vi "Joystick ReMap.vi"(2 "Deadband Size":dbl=0.02 min=-1.0 max=1.0 step=0.01, 3 "Raw Value":dbl) -> (0 "Modified Value (x^2)":dbl, 1 "Modified Value":dbl)   [LabVIEW 2014]
panel:
  # "The value entered here will be applied to both positive\nand negative values, so in a literal sense it is 1/2 the deadband\nsize, centered about zero."
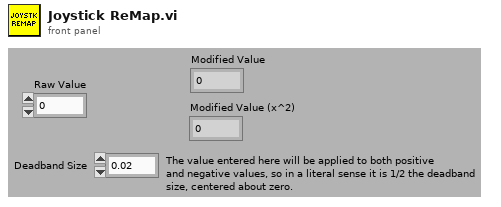
[diagram p1: front panel]
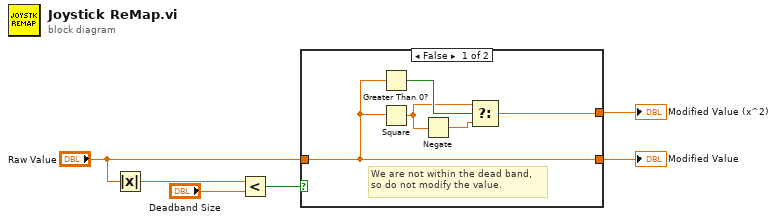
[diagram p0: block diagram]
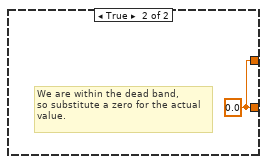
[diagram p2: hidden frame]
diagram:
  n1 = Absolute Value(x="Raw Value") -> (abs(x)=w5:dbl)
  n2 = Less?(x=w5, y="Deadband Size") -> (x < y?=w4:bool)
  n3 = case shown="False" w4 {
    tunnel: [w11 w12] -> w3
    tunnel: "Raw Value" -> [w11 _]
    tunnel: [w7 w12] -> w1
    frame False {
      # "We are not within the dead band,\nso do not modify the value."
      n4 = Greater Than 0?(x=w11) -> (x > 0?=w10:bool)
      n5 = Square(x=w11) -> (x^2=w8:dbl)
      n6 = Negate(x=w8) -> (-x=w9:dbl)
      n7 = Select(t=w8, s=w10, f=w9) -> (s? t:f=w7:dbl)
    }
    frame True {
      w12 = 0.0 ("Raw Value")
      # "We are within the dead band,\nso substitute a zero for the actual\nvalue."
    }
  }
  "Modified Value" <- w3
  "Modified Value (x^2)" <- w1
